vi "Exemple_Preprocessing_RobustScaler.vi"() -> ()   [LabVIEW 2020]
uses:
  Objet/6 - Datasets Transformation/6.3 - Processing Data/RobustScaler/RobustScaler.lvclass
panel:
  in  "y":string[][](array[string])
  in  "X":string[][](array[string])=[["1", "-2", "2"], ["-2", "1", "3"], ["4", "1", "-2"]]
  out "Data":T1
  out "error out":errorcluster
  in  "error in":errorcluster caption="entrée d'erreur"
  in  "RobustScaler":T2={"with_centering"=TRUE, "with_scaling"=TRUE, "quantile_range"={"q_min"=25.0, "q_max"=75.0}, "copy"=TRUE}
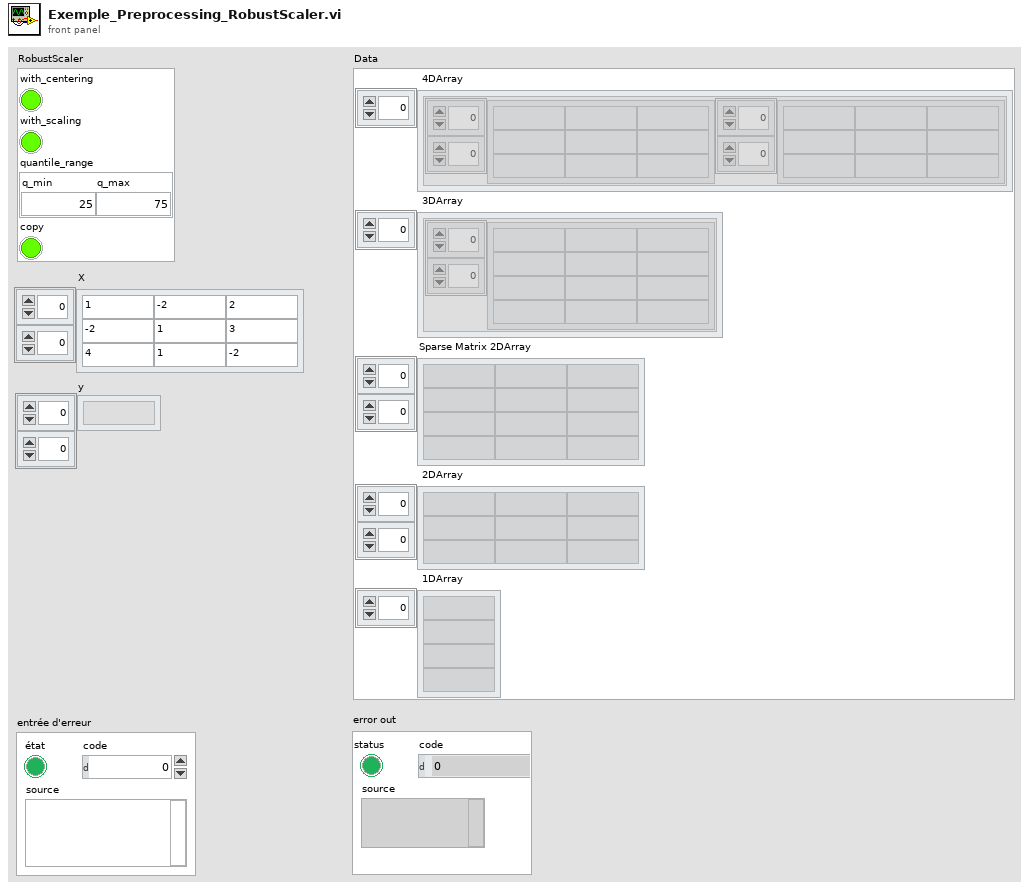
[diagram p1: front panel]
types:
  T1 = cluster{" 4DArray":cluster{"1":string[][], "2":string[][]}[], " 3DArray":cluster{"Tableau":string[][]}[], "Sparse Matrix 2DArray":string[][], " 2DArray":string[][], " 1DArray":string[]}
  T2 = cluster{"with_centering":bool, "with_scaling":bool, "quantile_range":cluster{"q_min":dbl, "q_max":dbl}, "copy":bool}
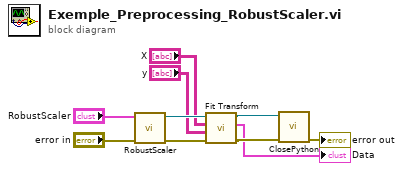
[diagram p0: block diagram]
diagram:
  n1 = call "RobustScaler.vi"("error in (no error)"="error in", "RobustScaler"="RobustScaler") -> ("error out"=w8:errorcluster, "RobustScaler.lvclass"=w7:refnum<class "RobustScaler.lvclass">)  [unwired: 8 in]
  n2 = call-dynamic "Fit Transform.vi"("error in (no error)"=w8, "y"="y", "X"="X", "RobustScaler.lvclass"=w7) -> ("error out"=w3:errorcluster, "Data"=→"Data":T1, "RobustScaler.lvclass"=w4:refnum<class "RobustScaler.lvclass">)  [unwired: 5 in]
  n3 = call-dynamic "ClosePython.vi"("error in (no error)"=w3, "Scikit-learn en entrée"=w4) -> ("error out"=→"error out":errorcluster)  [unwired: 8 in, 1 out]
